vi "Create Function String (List).vi"(8 "error in (no error)":errorcluster, 9 "Element (1: 1)":i32(ring)=1 items=["1"=1, "2"=2, "3"=3], 10 "Function (0: U)":i32(ring) items=["U", "I", "P", "PHIU", "PHII", "UHDF", "IHDF", "PHDF"], 11 "VISA resource name":refnum<visa-resource-name>) -> (0 "error out":errorcluster, 2 "Function String":string, 3 "VISA resource name out":refnum<visa-resource-name>)   [LabVIEW 2016, in "Yokogawa WT300 Series.lvlib"]
doc: "Create a list data function string"
uses:
  Yokogawa WT300 Series.lvlib
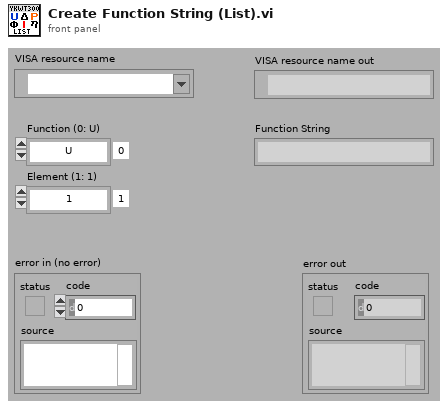
[diagram p1: front panel]
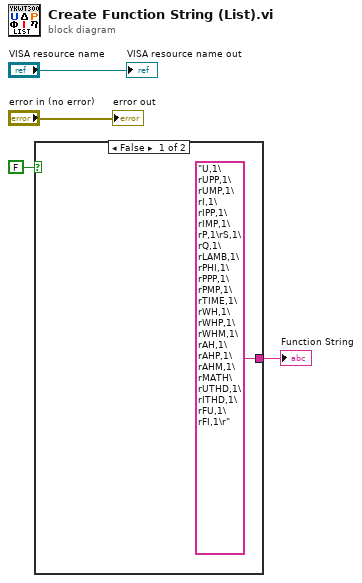
[diagram p0: block diagram]
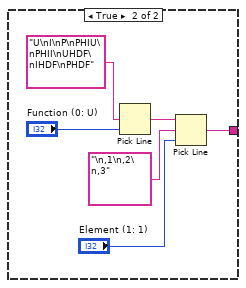
[diagram p2: hidden frame]
diagram:
  n1 = case shown="False" FALSE {
    tunnel: ["U,1\rUPP,1\rUMP,1\rI,1\rIPP,1\rIMP,1\rP,1\rS,1\rQ,1\rLAMB,1\rPHI,1\rPPP,1\rPMP,1\rTIME,1\rWH,1\rWHP,1\rWHM,1\rAH,1\rAHP,1\rAHM,1\rMATH\rUTHD,1\rITHD,1\rFU,1\rFI,1\r" ("concatenated string") w6] -> w2
    frame False {
    }
    frame True {
      n2 = Pick Line ("ライン選択")(multi-line string="U\nI\nP\nPHIU\nPHII\nUHDF\nIHDF\nPHDF" ("複数行文字列"), line index="Function (0: U)") -> (output string=w8:string)  [unwired: 1 in]
      n3 = Pick Line ("ライン選択")(string ("")=w8, multi-line string="\n,1\n,2\n,3" ("複数行文字列"), line index="Element (1: 1)") -> (output string=w6:string)
    }
  }
  "Function String" <- w2
  "VISA resource name out" <- "VISA resource name"
  "error out" <- "error in (no error)"
